vi "실습 3-2 난수 맞추기.vi"() -> ()   [LabVIEW 2014]
panel:
  out "가장 가까운 정수값":dbl
  out "x+1":i32
  in  "숫자형":dbl min=0.0 max=1000.0 step=1.0
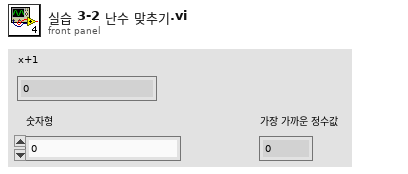
[diagram p1: front panel]
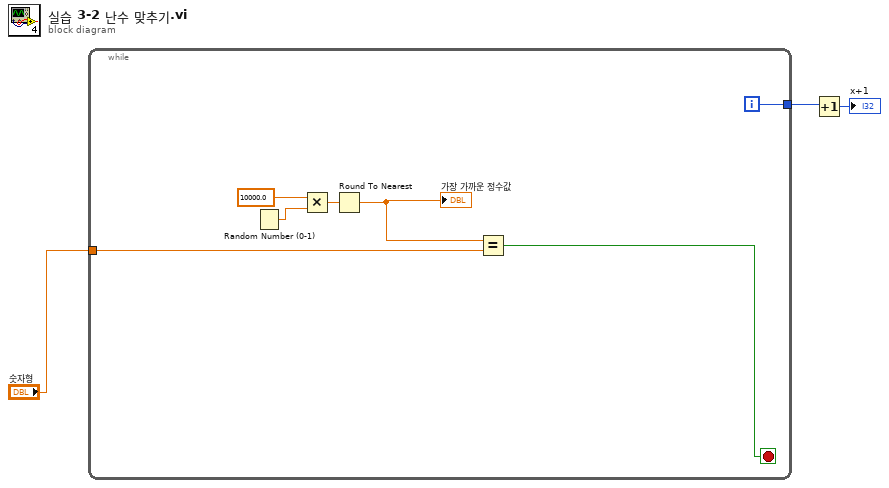
[diagram p0: block diagram]
diagram:
  n1 = while {
    tunnel: [w6] -> w3
    tunnel: "숫자형" -> [w4]
    i -> [w6]
    stop <- w7 stop-if-true
    n2 = Random Number (0-1)() -> (number: 0 to 1=w10:dbl)
    n3 = Multiply(x=10000.0, y=w10) -> (x*y=w8:dbl)
    n4 = Round To Nearest(number=w8) -> (nearest integer value=w5:dbl)
    "가장 가까운 정수값" <- w5
    n5 = Equal?(x=w5, y=w4) -> (x = y?=w7:bool)
  }
  n6 = Increment(x=w3) -> (x+1=→"x+1":i32)
